vi "Align 1 + N Waveforms (continuous).vi"(4 "interpolation":bool=TRUE, 6 "FIR filter specifications":T1={"alias rejection (dB)"=120.0, "normalized bandwidth"=0.4536} {"normalized bandwidth" format="%.4f"; "alias rejection (dB)" format="%.2f"}, 7 "reset":bool, 8 "error in (no error)":errorcluster, 9 "interpolation mode":u16(ring)=1 items=["coerce", "linear", "spline", "FIR filter"], 10 "waveforms in":waveform(dbl)[](array[waveform]), 11 "waveform in":waveform(dbl)) -> (0 "error out":errorcluster, 2 "aligned waveforms out":waveform(dbl)[](array[waveform]), 3 "aligned waveform out":waveform(dbl))   [LabVIEW 2020, in "NI_MAPro.lvlib"]
doc: "Performs element-wise alignment of waveforms and returns the aligned waveforms. The data types you wire to the waveform inputs determine the polymorphic instance to use."
uses:
  NI_MAPro.lvlib
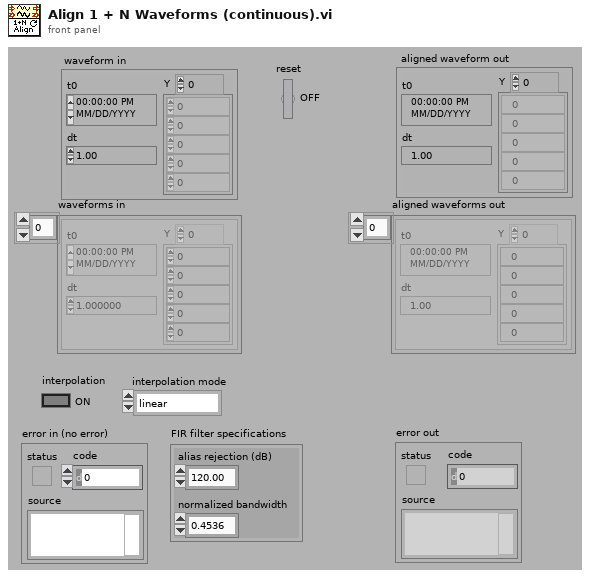
[diagram p1: front panel]
types:
  T1 = cluster{"alias rejection (dB)":dbl, "normalized bandwidth":dbl}
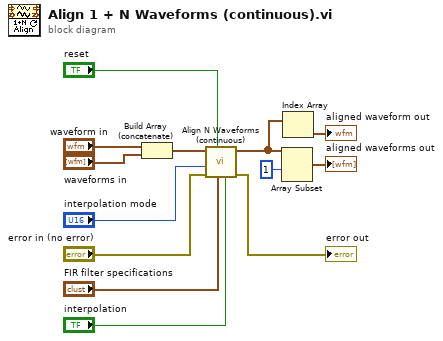
[diagram p0: block diagram]
diagram:
  n1 = Build Array (concatenate)("waveform in", "waveforms in") -> (w13:waveform(dbl)[])
  n2 = call "Align N Waveforms (continuous).vi"("interpolation"="interpolation", "FIR filter specifications"="FIR filter specifications", "reset"="reset", "error in (no error)"="error in (no error)", "interpolation mode"="interpolation mode", "waveforms in"=w13) -> ("error out"=→"error out":errorcluster, "waveforms out"=w10:waveform(dbl)[])  [unwired: 4 in]
  n3 = Array Subset(array=w10, index=1) -> (→"aligned waveforms out":waveform(dbl)[])  [unwired: 1 in]
  n4 = Index Array(array=w10) -> (element=→"aligned waveform out":waveform(dbl))  [unwired: 1 in]
